vi "Field to Robot Coords.vi"(9 "gyro":dbl, 10 "Joystick y":dbl, 11 "Joystick x":dbl) -> (2 "robot y":dbl, 3 "robot x":dbl)   [LabVIEW 2014]
panel:
  in  "negate y":bool
  in  "negate x":bool
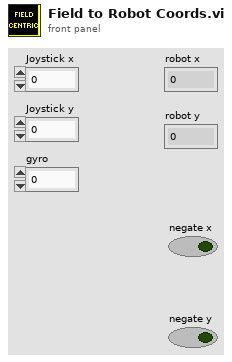
[diagram p1: front panel]
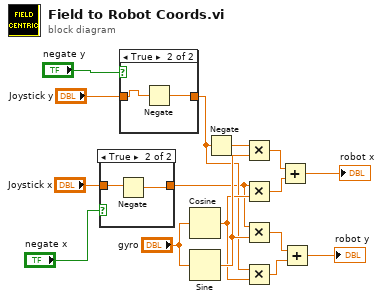
[diagram p0: block diagram]
diagram:
  n1 = case shown="True" "negate x" {
    tunnel: "Joystick x" -> [w17 w19]
    tunnel: [w17 w18] -> w3
    frame False {
    }
    frame True {
      n2 = Negate(x=w19) -> (-x=w18:dbl)
    }
  }
  n3 = case shown="True" "negate y" {
    tunnel: "Joystick y" -> [w20 w22]
    tunnel: [w20 w21] -> w5
    frame False {
    }
    frame True {
      n4 = Negate(x=w22) -> (-x=w21:dbl)
    }
  }
  n5 = Cosine(x="gyro") -> (cos(x)=w13:dbl)
  n6 = Sine(x="gyro") -> (sin(x)=w14:dbl)
  n7 = Negate(x=w5) -> (-x=w12:dbl)
  n8 = Multiply(x=w12, y=w14) -> (x*y=w8:dbl)
  n9 = Multiply(x=w3, y=w13) -> (x*y=w9:dbl)
  n10 = Multiply(x=w3, y=w14) -> (x*y=w10:dbl)
  n11 = Multiply(x=w5, y=w13) -> (x*y=w11:dbl)
  n12 = Add(x=w8, y=w9) -> (x+y=→"robot x":dbl)
  n13 = Add(x=w10, y=w11) -> (x+y=→"robot y":dbl)
